vi "VHMI-recieveConnectionInfo.vi"(8 "error in (no error)":errorcluster, 10 "connection status":T1, 11 "VDH-VNA_data_handler in":refnum<class "VDH-VNA_data_handler.lvclass">) -> (0 "error out":errorcluster, 3 "VDH-VNA_data_handler out":refnum<class "VDH-VNA_data_handler.lvclass">)   [LabVIEW 2020, in "VDH-VNA_data_handler.lvlib" / "VDH-VNA_data_handler.lvclass"]
uses:
  VDH-VNA_data_handler.lvclass
  hardware_manager/VHM-VNA_Hardware_Manager/VHM-VNA_Hardware_Manager/VHM-connection_status.ctl
  hardware_manager/VHM-VNA_Hardware_Manager/VHM-VNA_Hardware_Manager/VHM-VNA_Hardware_Manager.lvclass
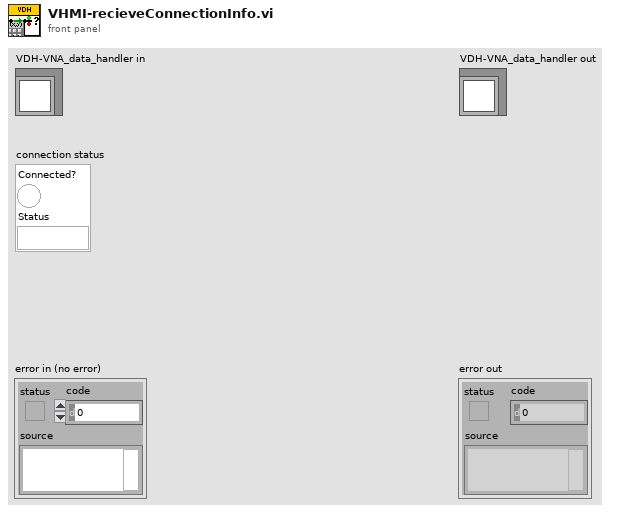
[diagram p1: front panel]
types:
  T1 = typedef "VHM-VNA_Hardware_Manager.lvlib/VHM-VNA_Hardware_Manager.lvclass/VHM-connection_status.ctl" = cluster{"Connected?":bool, "Status":string}
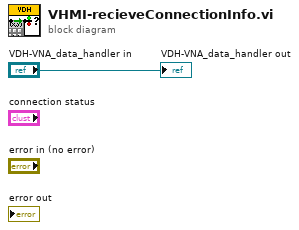
[diagram p0: block diagram]
diagram:
  "VDH-VNA_data_handler out" <- "VDH-VNA_data_handler in"
